vi "WriteDataToLabVIEWINI.vi"(8 "error in (no error)":errorcluster, 11 "INI Data":T1={"Show Terminals?"=FALSE, "Text"={"Font"="", "Alignment"=0, "Size"=0}, "3rd party Templates"={"Store 3rd party Templates?"=FALSE, "Folder Name"=""}, "Merge user layers on commit"=FALSE, "Body Text"={"Line 1 text"="", "Line 2 text"="", "Line 3 text"="", "Line 4 text"="", "Line 1 color"=0, "Line 2 color"=0, "Line 3 color"=0, "Line 4 color"=0, "Body Text Spec"={"Font"="", "Alignment"=0, "Size"=3}, "Center text vertically"=FALSE, "Capitalize Text"=FALSE}, "Fill Color"=0, "Edge Color"=0, "Tab"=0, "Tool"=enum."Ellipse", "Disable Layers?"=FALSE} {"Body Text"."Body Text Spec"."Alignment" items=["left", "center", "right"]; "Text"."Alignment" items=["left", "center", "right"]}) -> (0 "error out":errorcluster)   [LabVIEW 2021]
uses:
  <resource>/plugins/NIIconEditor/Controls/INI.ctl
  <vilib>/LabVIEW Icon API/lv_icon/Controls/Font.ctl
  <vilib>/LabVIEW Icon API/lv_icon/Controls/Alignment.ctl
  <resource>/plugins/NIIconEditor/Controls/Font Size.ctl
  <vilib>/LabVIEW Icon API/lv_icon/Controls/BodyText.ctl
  <vilib>/LabVIEW Icon API/lv_icon/Controls/IEColor.ctl
  <resource>/plugins/NIIconEditor/Controls/Tools.ctl
  <resource>/plugins/NIIconEditor/Controls/Pen.ctl
  <resource>/plugins/NIIconEditor/Controls/Line.ctl
  <resource>/plugins/NIIconEditor/Controls/Dropper.ctl
  <resource>/plugins/NIIconEditor/Controls/Fill.ctl
  <resource>/plugins/NIIconEditor/Controls/IERect.ctl
  <resource>/plugins/NIIconEditor/Controls/FRect.ctl
  <resource>/plugins/NIIconEditor/Controls/Circle.ctl
  <resource>/plugins/NIIconEditor/Controls/FCircle.ctl
  <resource>/plugins/NIIconEditor/Controls/Rubber.ctl
  <resource>/plugins/NIIconEditor/Controls/Text.ctl
  <resource>/plugins/NIIconEditor/Controls/Selection.ctl
  <resource>/plugins/NIIconEditor/Controls/Move.ctl
  <resource>/dialog/lvconfig.llb/LV Config Write String.vi
  <resource>/dialog/lvconfig.llb/LV Config Write Color.vi
  <resource>/dialog/lvconfig.llb/LV Config Write Boolean.vi
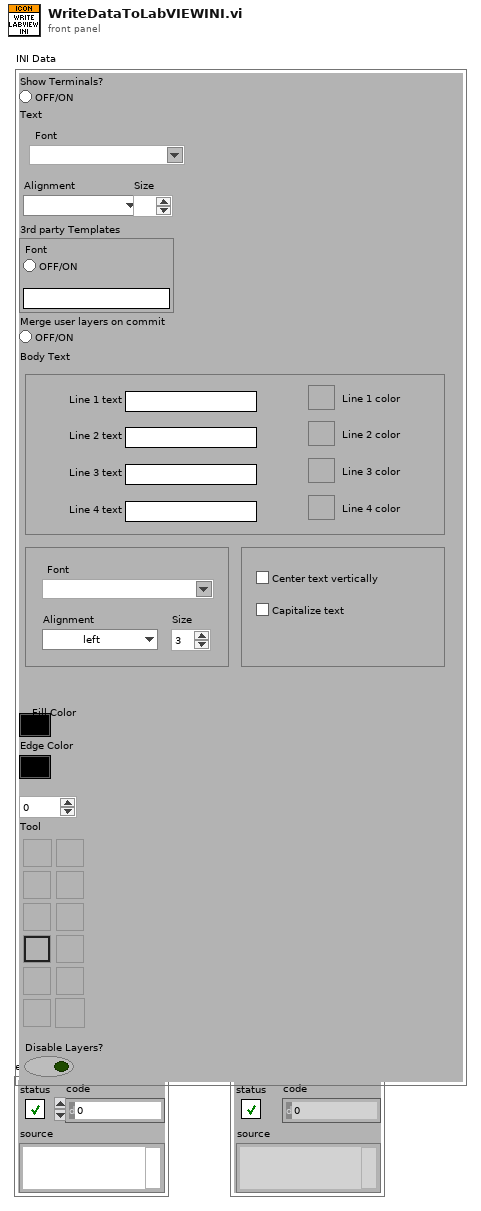
[diagram p1: front panel]
types:
  T1 = typedef "INI.ctl" = cluster{"Show Terminals?":bool, "Text":cluster{"Font":T2, "Alignment":T3, "Size":T4}, "3rd party Templates":cluster{"Store 3rd party Templates?":bool, "Folder Name":string}, "Merge user layers on commit":bool, "Body Text":T5, "Fill Color":T6, "Edge Color":T6, "Tab":u16, "Tool":T7, "Disable Layers?":bool}
  T2 = typedef "Font.ctl" = string
  T3 = typedef "Alignment.ctl" = u16
  T4 = typedef "Font Size.ctl" = u8
  T5 = typedef "BodyText.ctl" = cluster{"Line 1 text":string, "Line 2 text":string, "Line 3 text":string, "Line 4 text":string, "Line 1 color":u32, "Line 2 color":u32, "Line 3 color":u32, "Line 4 color":u32, "Body Text Spec":cluster{"Font":T2, "Alignment":T3, "Size":u8}, "Center text vertically":bool, "Capitalize Text":bool}
  T6 = typedef "IEColor.ctl" = u32
  T7 = typedef "Tools.ctl" = enum32{"Pencil", "Line", "Dropper", "Fill", "Rectangle", "Filled Rectangle", "Ellipse", "Filled Ellipse", "Eraser", "Text", "Select", "Move"}
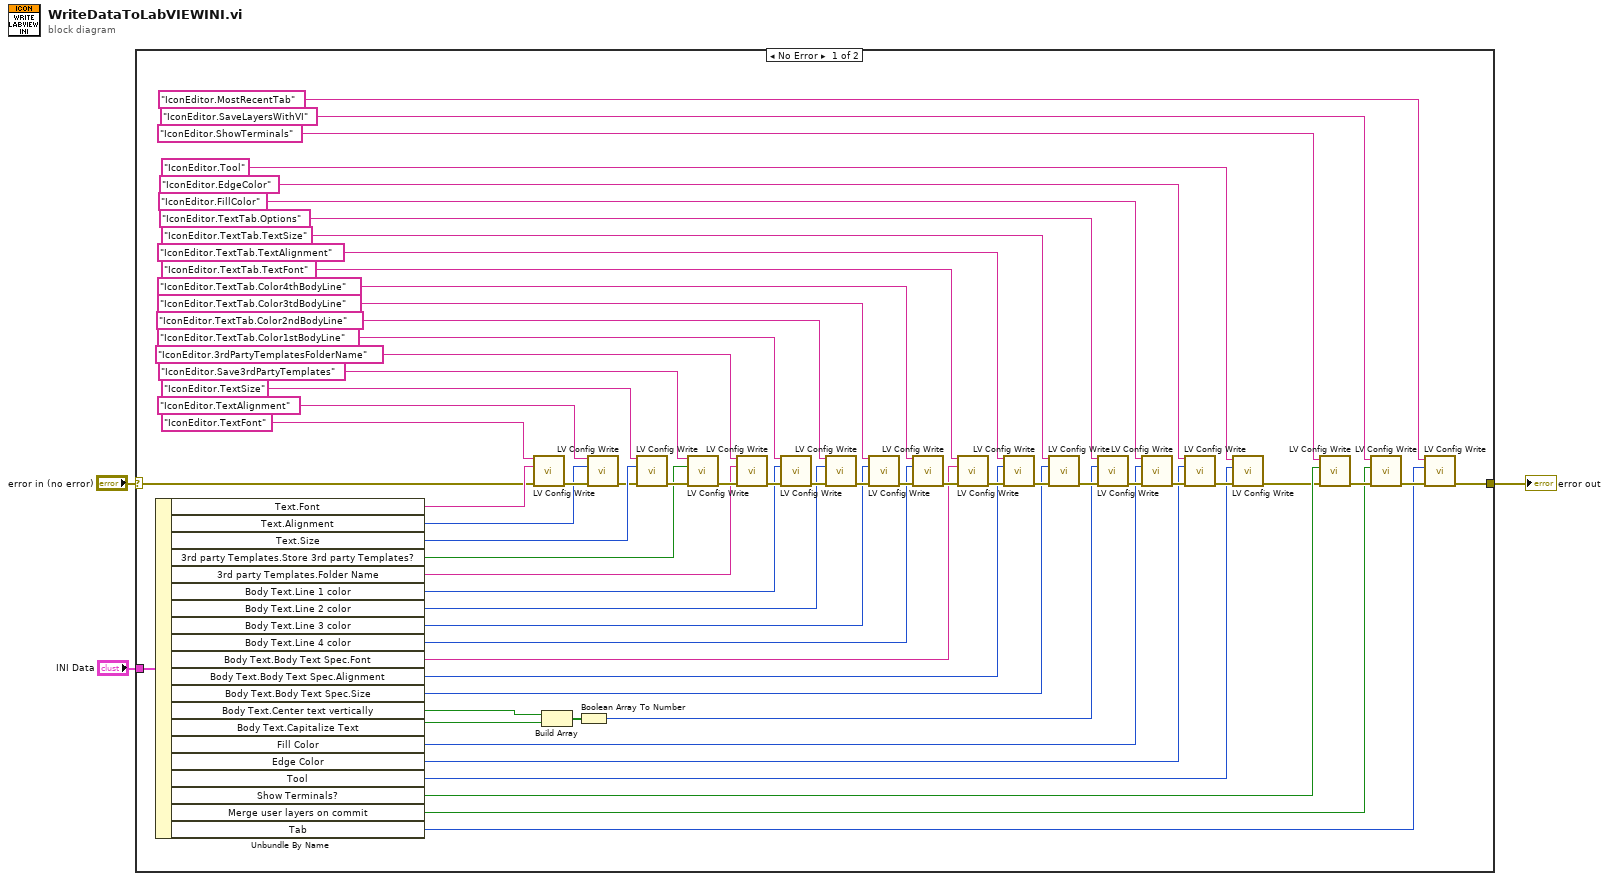
[diagram p0: block diagram]
diagram:
  n1 = case shown="No Error" "error in (no error)" {
    selector: "error in (no error)" -> [w6 w66]
    tunnel: [w5 w66] -> w2
    tunnel: "INI Data" -> [w65 _]
    frame No Error {
      n2 = Unbundle By Name(w65) -> ("Text.Font"=w64:T2, "Text.Alignment"=w61:T3, "Text.Size"=w59:T4, "3rd party Templates.Store 3rd party Templates?"=w55:bool, "3rd party Templates.Folder Name"=w52:string, "Body Text.Line 1 color"=w44:u32, "Body Text.Line 2 color"=w43:u32, "Body Text.Line 3 color"=w40:u32, "Body Text.Line 4 color"=w39:u32, "Body Text.Body Text Spec.Font"=w35:T2, "Body Text.Body Text Spec.Alignment"=w34:T3, "Body Text.Body Text Spec.Size"=w33:u8, "Body Text.Center text vertically"=w28:bool, "Body Text.Capitalize Text"=w29:bool, "Fill Color"=w19:T6, "Edge Color"=w18:T6, "Tool"=w15:T7, "Show Terminals?"=w14:bool, "Merge user layers on commit"=w10:bool, "Tab"=w7:u16)
      n3 = call-poly <resource>:"LV Config Write.vi"("error in (no error)"=w6, "value"=w64, "key"="IconEditor.TextFont") -> ("error out"=w62:errorcluster)  [unwired: 4 out]
      n4 = Build Array(w28, w29) -> (w27:bool[])
      n5 = Boolean Array To Number(Boolean array=w27) -> (number=w24:u32)
      n6 = call-poly <resource>:"LV Config Write.vi"("error in (no error)"=w62, "value"=w61, "key"="IconEditor.TextAlignment") -> ("error out"=w58:errorcluster)  [unwired: 4 out]
      n7 = call-poly <resource>:"LV Config Write.vi"("error in (no error)"=w58, "value"=w59, "key"="IconEditor.TextSize") -> ("error out"=w56:errorcluster)  [unwired: 4 out]
      n8 = call-poly <resource>:"LV Config Write.vi"("error in (no error)"=w56, "value"=w55, "key"="IconEditor.Save3rdPartyTemplates") -> ("error out"=w53:errorcluster)  [unwired: 4 out]
      n9 = call-poly <resource>:"LV Config Write.vi"("error in (no error)"=w53, "value"=w52, "key"="IconEditor.3rdPartyTemplatesFolderName") -> ("error out"=w50:errorcluster)  [unwired: 4 out]
      n10 = call-poly <resource>:"LV Config Write.vi"("error in (no error)"=w50, "value"=w44, "key"="IconEditor.TextTab.Color1stBodyLine") -> ("error out"=w49:errorcluster)  [unwired: 4 out]
      n11 = call-poly <resource>:"LV Config Write.vi"("error in (no error)"=w49, "value"=w43, "key"="IconEditor.TextTab.Color2ndBodyLine") -> ("error out"=w42:errorcluster)  [unwired: 4 out]
      n12 = call-poly <resource>:"LV Config Write.vi"("error in (no error)"=w42, "value"=w40, "key"="IconEditor.TextTab.Color3tdBodyLine") -> ("error out"=w41:errorcluster)  [unwired: 4 out]
      n13 = call-poly <resource>:"LV Config Write.vi"("error in (no error)"=w41, "value"=w39, "key"="IconEditor.TextTab.Color4thBodyLine") -> ("error out"=w38:errorcluster)  [unwired: 4 out]
      n14 = call-poly <resource>:"LV Config Write.vi"("error in (no error)"=w38, "value"=w35, "key"="IconEditor.TextTab.TextFont") -> ("error out"=w37:errorcluster)  [unwired: 4 out]
      n15 = call-poly <resource>:"LV Config Write.vi"("error in (no error)"=w37, "value"=w34, "key"="IconEditor.TextTab.TextAlignment") -> ("error out"=w36:errorcluster)  [unwired: 4 out]
      n16 = call-poly <resource>:"LV Config Write.vi"("error in (no error)"=w36, "value"=w33, "key"="IconEditor.TextTab.TextSize") -> ("error out"=w26:errorcluster)  [unwired: 4 out]
      n17 = call-poly <resource>:"LV Config Write.vi"("error in (no error)"=w26, "value"=w24, "key"="IconEditor.TextTab.Options") -> ("error out"=w23:errorcluster)  [unwired: 4 out]
      n18 = call-poly <resource>:"LV Config Write.vi"("error in (no error)"=w23, "value"=w19, "key"="IconEditor.FillColor") -> ("error out"=w22:errorcluster)  [unwired: 4 out]
      n19 = call-poly <resource>:"LV Config Write.vi"("error in (no error)"=w22, "value"=w18, "key"="IconEditor.EdgeColor") -> ("error out"=w17:errorcluster)  [unwired: 4 out]
      n20 = call-poly <resource>:"LV Config Write.vi"("error in (no error)"=w17, "value"=w15, "key"="IconEditor.Tool") -> ("error out"=w4:errorcluster)  [unwired: 4 out]
      n21 = call-poly <resource>:"LV Config Write.vi"("error in (no error)"=w4, "value"=w14, "key"="IconEditor.ShowTerminals") -> ("error out"=w12:errorcluster)  [unwired: 4 out]
      n22 = call-poly <resource>:"LV Config Write.vi"("error in (no error)"=w12, "value"=w10, "key"="IconEditor.SaveLayersWithVI") -> ("error out"=w9:errorcluster)  [unwired: 4 out]
      n23 = call-poly <resource>:"LV Config Write.vi"("error in (no error)"=w9, "value"=w7, "key"="IconEditor.MostRecentTab") -> ("error out"=w5:errorcluster)  [unwired: 4 out]
    }
    frame Error {
    }
  }
  "error out" <- w2
